vi "vector_vect2cord.vi"(11 "Vector":cluster{"R":dbl, "theta":dbl}) -> (3 "Coordinate":cluster{"X":dbl, "Y":dbl})   [LabVIEW 2011]
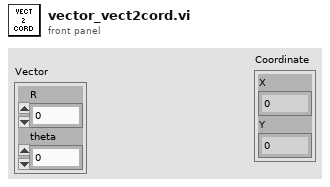
[diagram p1: front panel]
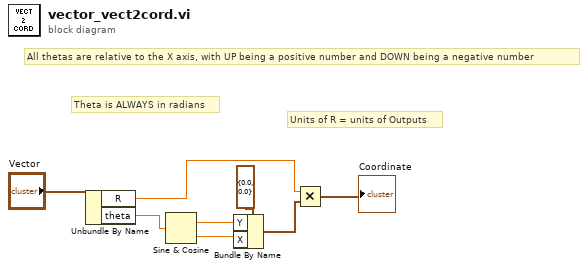
[diagram p0: block diagram]
diagram:
  # "Units of R = units of Outputs"
  # "Theta is ALWAYS in radians"
  # "All thetas are relative to the X axis, with UP being a positive number and DOWN being a negative number"
  n1 = Unbundle By Name("Vector") -> ("R"=w3:dbl, "theta"=w7:dbl)
  n2 = Sine & Cosine(0:w7) -> (1:w6:dbl, 2:w5:dbl)
  n3 = Bundle By Name(cluster=cluster{"X":dbl, "Y":dbl} {"X"=0.0, "Y"=0.0} ("Coordinate"), "Y"=w6, "X"=w5) -> (w1:cluster{"X":dbl, "Y":dbl})
  n4 = Multiply(x=w3, y=w1) -> (x*y=→"Coordinate":cluster{"X":dbl, "Y":dbl})
